vi "GET ATRIUM PHOTO.vi"(10 "Image In":T1, 11 "REFERENCES":T2) -> (2 "Image Out":T1)   [LabVIEW 2019]
uses:
  Controls/References Cluster.ctl
  <vilib>/userDefined/High Color/IMAQdx.ctl
  Controls/Custom Calendar/Custom Calendar.xctl
  <vilib>/vision/Image Controls.llb/IMAQ Image.ctl
  <vilib>/regexp/Match Regular Expression.xnode
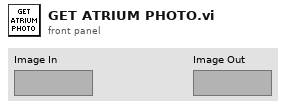
[diagram p1: front panel]
types:
  T1 = typedef "IMAQ Image.ctl" = refnum<image>
  T2 = typedef "References Cluster.ctl" = cluster{"MAIN PAGES":refnum<vi>, "ADD/EDIT ITEM REFERENCES":cluster{"Identifier":refnum<vi>, "BYU ICN #":refnum<vi>, "Item Description":refnum<vi>, "Comments":refnum<vi>, "Checked Out Date":refnum<vi>, "Due Date":refnum<vi>, "Check Out Location":refnum<vi>, "Reminder Count":refnum<vi>, "Most Recent Reminder Date":refnum<vi>, "BYU ID #":refnum<vi>, "Building/Room":refnum<vi>, "Location in Room":refnum<vi>, "Manual":refnum<vi>, "Manufacturer":refnum<vi>, "Model #":refnum<vi>, "Serial #":refnum<vi>, "Date Acquired":refnum<vi>, "ADD/EDIT ITEM LABEL":refnum<vi>, "ARCHIVE ITEM":refnum<vi>, "Archive Item Inputs":refnum<vi>, "Reminder Notes":refnum<vi>}, "ADD/EDIT USER REFERENCES":cluster{"BYU ID # (##-###-####)":refnum<vi>, "First Name":refnum<vi>, "Last Name":refnum<vi>, "Phone Number (###-###-####)":refnum<vi>, "Email":refnum<vi>, "Department":refnum<vi>, "Graduation Status":refnum<vi>, "Anticipated Graduation Year":refnum<vi>, "Credit Score":refnum<vi>, "Date Added":refnum<vi>, "Graduation Clearance Date":refnum<vi>, "Picture File Name":refnum<vi>, "ADD/EDIT USER LABEL":refnum<vi>, "Department Map":refnum<vi>, "Status Map":refnum<vi>, "Anticipated Graduation Year Map":refnum<vi>, "User Agreement":refnum<vi>, "User Comments":refnum<vi>, "Camera":refnum<vi>}, "RETURN ITEM REFERENCES":cluster{"Item or Person:":refnum<vi>, "Search Return Results":refnum<vi>, "What are you searching for?":refnum<vi>}, "SEARCH DATABASE REFERENCES":cluster{"What to Search For:":refnum<vi>, "Where to Search":refnum<vi>, "Column to Search In":refnum<vi>, "Column to Sort By":refnum<vi>, "Search Database Results":refnum<vi>, "Inventory Column Selector":refnum<vi>, "User Column Selector":refnum<vi>, "Inventory Archive Column Selector":refnum<vi>, "User Archive Column Selector":refnum<vi>, "Sales Tracking Column Selector":refnum<vi>, "Checked In Archive Column Selector":refnum<vi>, "Restore User":refnum<vi>, "Date Range":refnum<vi>, "Dates Less Than":refnum<vi>, "Dates Greater Than":refnum<vi>, "Search Print Receipt":refnum<vi>}, "USER ITEMS REFERENCES":cluster{"USER'S INFORMATION":refnum<vi>, "User's Checked Out Items":refnum<vi>, "User Info Comments":refnum<vi>, "SEE USER INFO COMMENTS":refnum<vi>}, "EDIT ITEMS REFERENCES":cluster{"New Check Out Location":refnum<vi>, "Items to Edit":refnum<vi>, "Edit Items Due Date":refnum<vi>, "New Reminder Notes":refnum<vi>, "New Item Description":refnum<vi>}, "CHECK OUT ITEMS REFERENCES":cluster{"Enter Item:":refnum<vi>, "Check Out Items Due Date":refnum<vi>, "Check Out Location":refnum<vi>, "Items to be Checked Out":refnum<vi>, "Possible Items":refnum<vi>}, "TRANSFER ITEMS REFERENCES":cluster{"Search Parameter":refnum<vi>, "What to Match":refnum<vi>, "Matching Individuals":refnum<vi>, "Items to be Transferred":refnum<vi>}, "SETTINGS REFERENCES":cluster{"PSC Database Settings":refnum<vi>, "PSC Sales Item Spreadsheet":refnum<vi>}, "PSC SALES REFERENCES":cluster{"BYU ID CARD #":refnum<vi>, "Sale Description":refnum<vi>, "Scan or Enter Item Name":refnum<vi>, "Items to be Sold":refnum<vi>, "Grand Total":refnum<vi>, "Item List":refnum<vi>}}
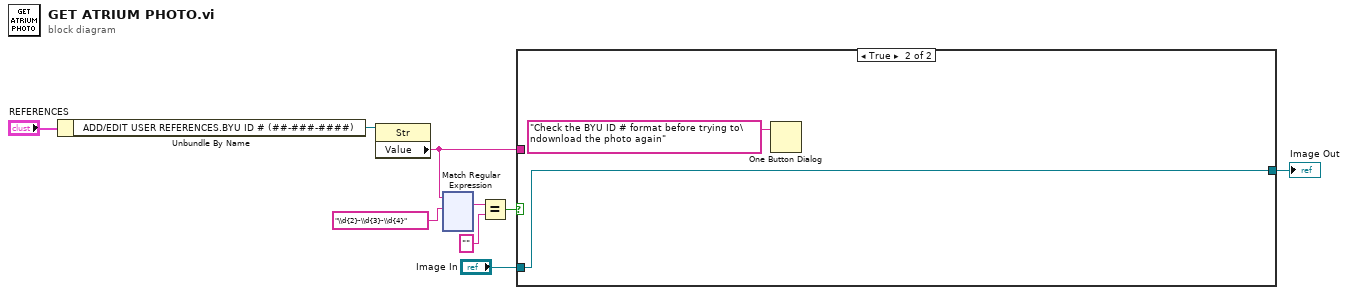
[diagram p0: block diagram]
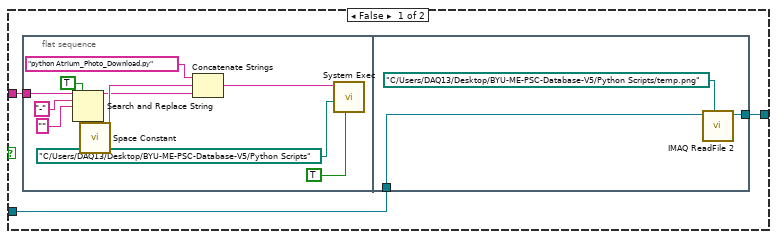
[diagram p2: hidden frame]
diagram:
  n1 = Unbundle By Name("REFERENCES") -> ("ADD/EDIT USER REFERENCES.BYU ID # (##-###-####)"=w8:refnum<vi>)
  n2 = property class="Str"(reference=w8) -> ("Value"=w3:string)  [unwired: 1 in, 2 out]
  n3 = xnode "Match Regular Expression"("input string"=w3, "regular expression"="\\d{2}-\\d{3}-\\d{4}") -> ("whole match"=w6:string)  [unwired: 4 in, 4 out]
  n4 = Equal?(x=w6, y="") -> (x = y?=w4:bool)
  n5 = case shown="True" w4 {
    tunnel: w3 -> [w12 _]
    tunnel: "Image In" -> [w11 w26]
    tunnel: [w10 w26] -> w1
    frame False {
      n6 = flat-sequence {
        tunnel: w12 -> [w13]
        tunnel: w11 -> [w24]
        tunnel: [w23] -> w10
        frame #0 {
          n7 = Search and Replace String(replace all?=TRUE ("replace all? (F)"), input string=w13, search string="-", replace string="" ("replace string (\"\")")) -> (result string=w17:string)  [unwired: 4 in, 3 out]
          n8 = call <vilib>:"Space Constant.vi"() -> ("String"=w18:string)
          n9 = Concatenate Strings("python Atrium_Photo_Download.py" ("command line"), w18, w17) -> (w16:string)
          n10 = call <vilib>:"System Exec.vi"("run minimized? (F)"=TRUE, "working directory"=path "C:/Users/DAQ13/Desktop/BYU-ME-PSC-Database-V5/Python Scripts" ("File Path"), "command line"=w16) -> ()  [unwired: 5 in, 4 out]
        }
        frame #1 {
          n11 = call "IMAQ ReadFile 2"("File Path"=path "C:/Users/DAQ13/Desktop/BYU-ME-PSC-Database-V5/Python Scripts/temp.png", "Image"=w24) -> ("Image Out"=w23:T1)  [unwired: 5 in, 4 out]
        }
      }
    }
    frame True {
      n12 = One Button Dialog(message="Check the BYU ID # format before trying to\ndownload the photo again") -> ()  [unwired: 1 in, 1 out]
    }
  }
  "Image Out" <- w1
